vi "Drop Into MacroTree.vi"(0 "UI control refnums":T2, 1 "Index IN":i32, 5 "Source Tag":string, 7 "Source Text":string, 9 "Destination Tag":string, 11 "Error In":errorcluster, 12 "Drag Source":T1(ring)) -> (4 "Index OUT":i32, 14 "Any Error? OUT":bool, 15 "Error Out":errorcluster)   [LabVIEW 2012]
doc: "SciScan 1.2 160622"
uses:
  Custom Controls and Typedefs/Macro_MD_UI Control Refnums.ctl
  Custom Controls and Typedefs/Delete Button.ctl
  Custom Controls and Typedefs/Edit Button.ctl
  Custom Controls and Typedefs/Timing Estimate Cluster.ctl
  CommonResource VIs/Timing/Timing Indicator.ctl
  Custom Controls and Typedefs/Load from PSM Button.ctl
  CommonResource VIs/FormatTree&TableStyle_Commands.ctl
  Macro Loop Manager Module/SubVIs/Macro Execution and Timing_Commands.ctl
  SubVIs/FGV_MacroCore_Commands.ctl
panel:
  out "Specified tag is part of a Preset!":bool
  # "(hh:mm:ss)"
  # "(hh:mm:ss)"
  # "(hh:mm:ss)"
  # "(hh:mm:ss)"
  # "(hh:mm:ss)"
  # "(hh:mm:ss)"
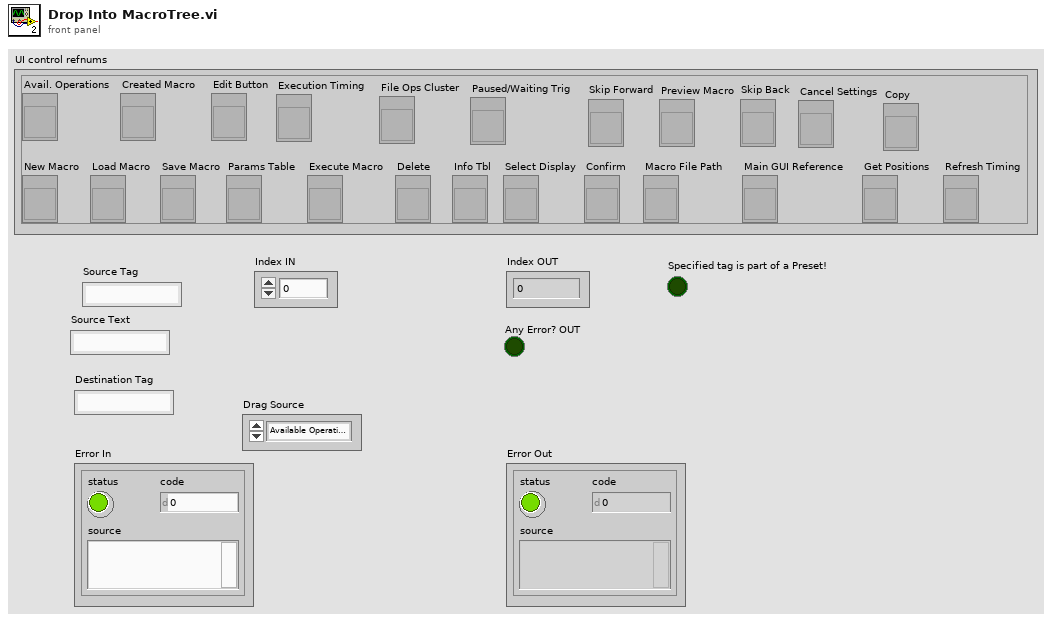
[diagram p1: front panel]
types:
  T1 = enum16{"Available Operations Tree", "Macro Tree"}
  T2 = typedef "Macro_MD_UI Control Refnums.ctl" = cluster{"Avail. Operations":refnum<vi>, "Created Macro":refnum<vi>, "Load Macro":refnum<vi>, "Save Macro":refnum<vi>, "Params Table":refnum<vi>, "Delete":refnum<vi>, "Edit Button":refnum<vi>, "Execute Macro":refnum<vi>, "Info Tbl":refnum<vi>, "Execution Timing":refnum<vi>, "Select Display":refnum<vi>, "File Ops Cluster":refnum<vi>, "Paused/Waiting Trig":refnum<vi>, "Confirm":refnum<vi>, "New Macro":refnum<vi>, "Preview Macro":refnum<vi>, "Skip Forward":refnum<vi>, "Skip Back":refnum<vi>, "Macro File Path":refnum<vi>, "Main GUI Reference":refnum<vi>, "Cancel Settings":refnum<vi>, "Get Positions":refnum<vi>, "Copy":refnum<vi>, "Refresh Timing":refnum<vi>}
  T3 = typedef "Macro Execution and Timing_Commands.ctl" = enum16{"Initialize (Update FGV & Rst Idx)", "Run", "EstimateTime", "Preview", "Update Macro array (Idx Unchanged)", "Update Index", "Clear Timing Info"}
  T4 = typedef "FormatTree&TableStyle_Commands.ctl" = enum16{"Colour Row", "Uncolour Row", "Bold Row", "Unbold Row", "Clear", "UpdateVisibleRows"}
  T5 = typedef "FGV_MacroCore_Commands.ctl" = enum16{"Initialize", "Get Array", "Load macro from file", "Insert Item", "Insert at End", "Edit Parameter String", "Delete instruction", "Move Items", "Save", "SaveAs", "UpdateInfoTable", "Edit Settings File", "New Macro", "Read Temp File", "Delete Multiple"}
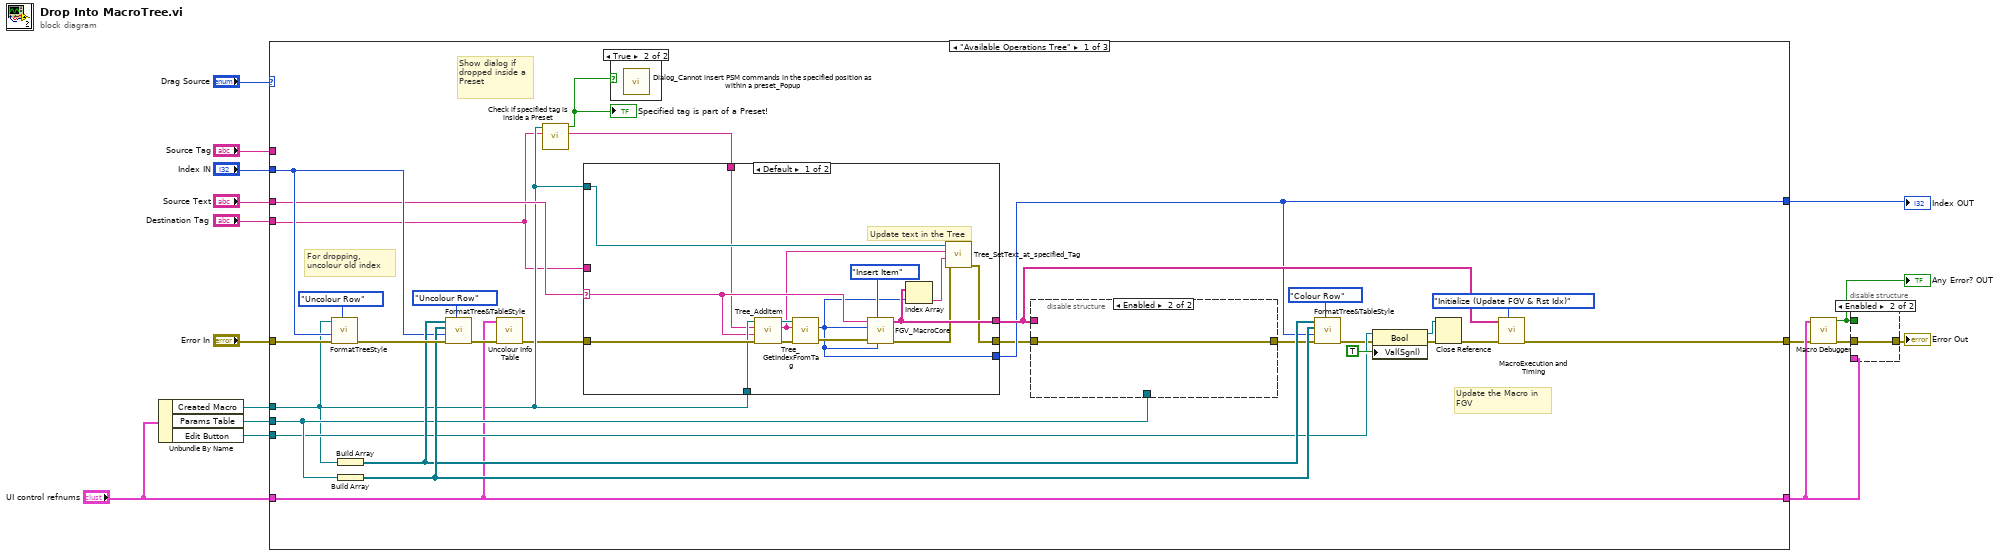
[diagram p0: block diagram]
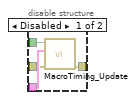
[diagram p2: hidden frame]
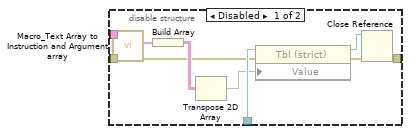
[diagram p4: hidden frame]
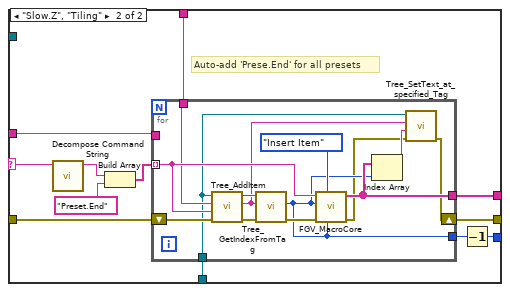
[diagram p5: hidden frame]
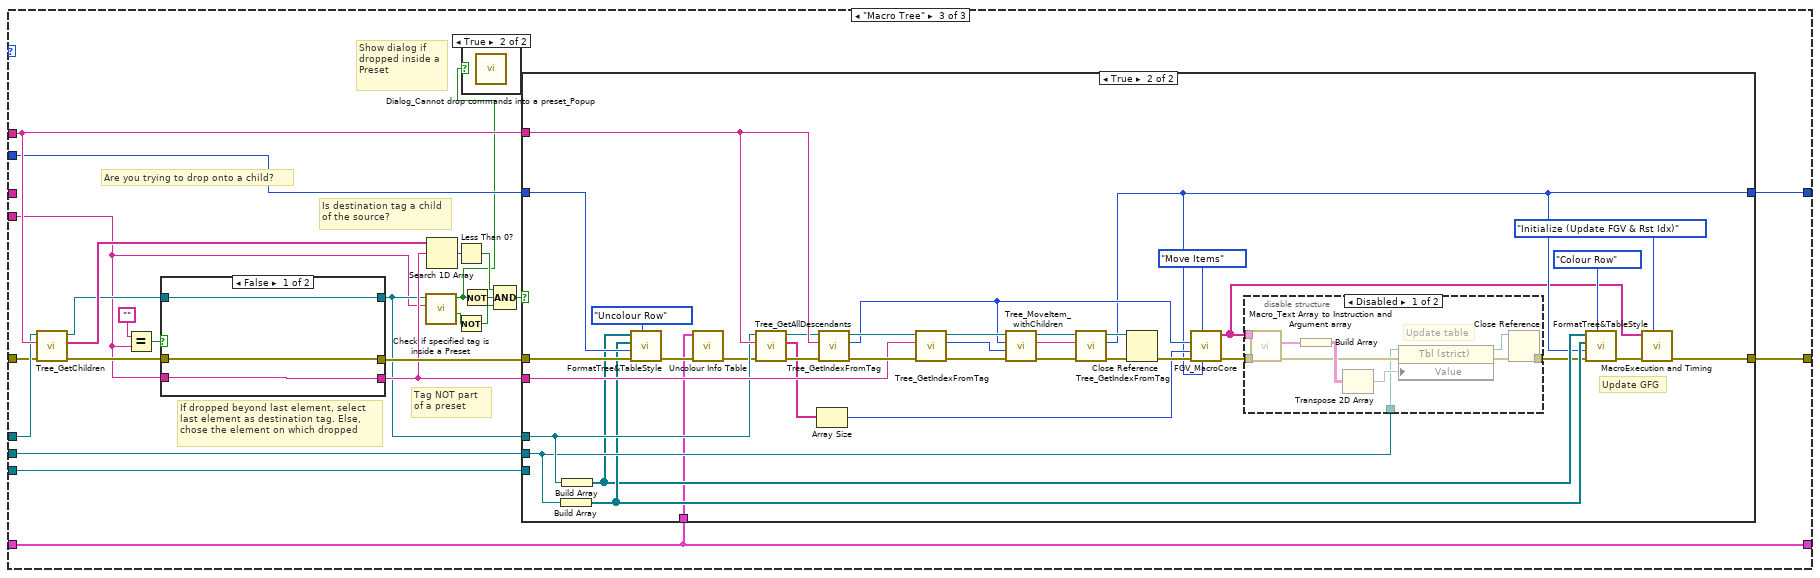
[diagram p7: hidden frame]
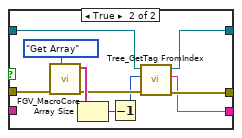
[diagram p9: hidden frame]
diagram:
  n1 = Unbundle By Name("UI control refnums") -> ("Created Macro"=w7:refnum<vi>, "Params Table"=w8:refnum<vi>, "Edit Button"=w9:refnum<vi>)
  n2 = case shown="\"Available Operations Tree\"" "Drag Source" {
    tunnel: "Source Tag" -> [_ _ w120]
    tunnel: "UI control refnums" -> [w26 w98 w109]
    tunnel: "Destination Tag" -> [w20 _ w107]
    tunnel: "Error In" -> [w32 w99 w113]
    tunnel: "Index IN" -> [w33 w100 w119]
    tunnel: [w24 w100 w118] -> w11
    tunnel: w9 -> [w34 _ w117]
    tunnel: w8 -> [w35 _ w116]
    tunnel: w7 -> [w22 _ w114]
    tunnel: "Source Text" -> [w23 _ _]
    tunnel: [w25 w99 w115] -> w3
    tunnel: [w26 w98 w109] -> w5
    frame "Available Operations Tree" {
      # "Show dialog if dropped inside a Preset"
      # "Update the Macro in \nFGV"
      # "For dropping, uncolour old index"
      n3 = call "FormatTreeStyle.vi"("Format Command"=FormatTree&TableStyle_Commands."Uncolour Row", "Error In"=w32, "Row Index"=w33, "Tree Refnum"=w22) -> ("Error Out"=w39:errorcluster)  [unwired: 7 in]
      n4 = Build Array(w22) -> (w37:refnum<vi>[])
      n5 = Build Array(w35) -> (w38:refnum<vi>[])
      n6 = call "FormatTree&TableStyle.vi"("Format Command"=FormatTree&TableStyle_Commands."Uncolour Row", "Error In"=w39, "Row Index"=w33, "Array of Table references"=w38, "Array of Tree references"=w37) -> ("Error Out"=w36:errorcluster)  [unwired: 6 in]
      n7 = call "Uncolour Info Table.vi"("Error In"=w36, "UI control refnums"=w26) -> ("Error Out"=w18:errorcluster)  [unwired: 9 in]
      n8 = call "Check if specified tag is inside a Preset.vi"("Tag to check"=w20, "Tree Refnum"=w22) -> ("Tag to add new item"=w19:string, "Specified tag is part of a Preset?"=w21:bool)  [unwired: 6 in, 2 out]
      "Specified tag is part of a Preset!" <- w21
      n9 = case shown="Default" w23 {
        selector: w23 -> [w65 w73]
        tunnel: [w58 w83] -> w17
        tunnel: w18 -> [w67 w82]
        tunnel: w20 -> [_ w75]
        tunnel: w22 -> [w66 w76]
        tunnel: [w64 w81] -> w27
        tunnel: [w63 w78] -> w24
        tunnel: w19 -> [w60 w74]
        tunnel: w22 -> [w61 _]
        frame Default {
          # "Update text in the Tree"
          n10 = call "Tree_AddItem.vi"("Error In"=w67, "NEW String"=w65, "Tag at add position"=w60, "Tree Refnum"=w66) -> ("Error Out"=w70:errorcluster, "Added Item Tag"=w57:string, "Tree Refnum OUT"=w68:refnum<vi>)  [unwired: 5 in]
          n11 = call "Tree_GetIndexFromTag.vi"("Error In"=w70, "Tag IN"=w57, "Tree Refnum IN"=w68) -> ("Error Out"=w69:errorcluster, "Index OUT"=w63:i32)  [unwired: 6 in, 1 out]
          n12 = call "FGV_MacroCore.vi"("Final Index"=w63, "MacroFGV_Commands"=FGV_MacroCore_Commands."Insert Item", "Error In"=w69, "Start Index"=w63, "Macro Command or Info (String)"=w65) -> ("Error Out"=w59:errorcluster, "Macro String Array"=w64:string[])  [unwired: 2 in, 3 out]
          n13 = Index Array(array=w64, index=w63) -> (element=w62:string)
          n14 = call "Tree_SetText_at_specified_Tag.vi"("Error In"=w59, "New String IN"=w62, "Tag (whose string to be edited)"=w57, "Tree Refnum IN"=w61) -> ("Error Out"=w58:errorcluster)  [unwired: 6 in, 1 out]
        }
        frame "Slow.Z", "Tiling" {
          # "Auto-add 'Prese.End' for all presets"
          n15 = call "Decompose Command String.vi"("Command IN"=w73) -> ("Action"=w72:string)  [unwired: 7 in, 3 out]
          n16 = Build Array(w72, "Preset.End" ("element")) -> (w77:string[])
          n17 = for {
            tunnel: w76 -> [w90]
            tunnel: [w88] -> w81
            tunnel: [w87] -> w79
            tunnel: w77 -> [w93] mode=indexing
            shift-right: [w84] -> w83
            shift-left: w82 -> [w94]
            tunnel: w75 -> [_]
            tunnel: w74 -> [w92]
            n18 = call "Tree_AddItem.vi"("Error In"=w94, "NEW String"=w93, "Tag at add position"=w92, "Tree Refnum"=w90) -> ("Error Out"=w96:errorcluster, "Added Item Tag"=w89:string, "Tree Refnum OUT"=w91:refnum<vi>)  [unwired: 5 in]
            n19 = call "Tree_GetIndexFromTag.vi"("Error In"=w96, "Tag IN"=w89, "Tree Refnum IN"=w91) -> ("Error Out"=w95:errorcluster, "Index OUT"=w87:i32)  [unwired: 6 in, 1 out]
            n20 = call "FGV_MacroCore.vi"("Final Index"=w87, "MacroFGV_Commands"=FGV_MacroCore_Commands."Insert Item", "Error In"=w95, "Start Index"=w87, "Macro Command or Info (String)"=w93) -> ("Error Out"=w85:errorcluster, "Macro String Array"=w88:string[])  [unwired: 2 in, 3 out]
            n21 = Index Array(array=w88, index=w87) -> (element=w86:string)
            n22 = call "Tree_SetText_at_specified_Tag.vi"("Error In"=w85, "New String IN"=w86, "Tag (whose string to be edited)"=w89, "Tree Refnum IN"=w90) -> ("Error Out"=w84:errorcluster)  [unwired: 6 in, 1 out]
          }
          n23 = Decrement(x=w79) -> (x-1=w78:i32)
        }
      }
      n24 = case shown="True" w21 {
        frame False {
        }
        frame True {
          n25 = call "Dialog_Cannot insert PSM commands in the specified position as within a preset_Popup.vi"() -> ()  [unwired: 11 in, 1 out]
        }
      }
      n26 = disable-structure shown="Enabled" {
        disable-tunnel: w17 -> [w55 w56]
        disable-tunnel: w35 -> [w54 _]
        disable-tunnel: [w53 w56] -> w30
        disable-tunnel: w27 -> [w52 _]
        frame Disabled {
          n27 = call "Macro_Text Array to Instruction and Argument array.vi"("Error In"=w55, "Macro Array IN"=w52) -> ("Error Out"=w49:errorcluster, "Argument List (Txt)"=w48:string[])  [unwired: 7 in, 1 out]
          n28 = Build Array(w48) -> (w51:string[][])
          n29 = Transpose 2D Array(2D array=w51) -> (transposed array=w50:string[][])
          n30 = property class="Tbl (strict)"(reference=w54, error in=w49, "Value"=w50) -> (reference out=w46:refnum<vi>, error out=w47:errorcluster)
          n31 = Close Reference(reference=w46, error in (no error)=w47) -> (error out=w53:errorcluster)
        }
        frame Enabled {
        }
      }
      n32 = call "FormatTree&TableStyle.vi"("Format Command"=FormatTree&TableStyle_Commands."Colour Row", "Error In"=w30, "Row Index"=w24, "Array of Table references"=w38, "Array of Tree references"=w37) -> ("Error Out"=w31:errorcluster)  [unwired: 6 in]
      n33 = property class="Bool"(reference=w34, error in=w31, "Val(Sgnl)"=TRUE) -> (reference out=w43:refnum<vi>, error out=w44:errorcluster)
      n34 = Close Reference(reference=w43, error in (no error)=w44) -> (error out=w28:errorcluster)
      n35 = call "MacroExecution and Timing.vi"("MacroExecution and Timing Command"=Macro_Execution_and_Timing_Commands."Initialize (Update FGV & Rst Idx)" ("MacroExecution Command"), "Error In"=w28, "Macro IN"=w27) -> ("Error Out"=w25:errorcluster)  [unwired: 3 in, 5 out]
    }
    frame Default {
    }
    frame "Macro Tree" {
      # "Show dialog if dropped inside a Preset"
      # "Tag NOT part of a preset"
      # "Is destination tag a child\nof the source?"
      # "Are you trying to drop onto a child?"
      # "If dropped beyond last element, select\nlast element as destination tag. Else,\nchose the element on which dropped"
      n36 = call "Tree_GetChildren.vi"("Error In"=w113, "Parent Tag"=w120, "Tree Refnum IN"=w114) -> ("Error Out"=w112:errorcluster, "Children Tags"=w125:string[], "Tree Refnum OUT"=w111:refnum<vi>)  [unwired: 6 in]
      n37 = Equal?(x="", y=w107) -> (x = y?=w122:bool)
      n38 = case shown="False" w122 {
        tunnel: w112 -> [w128 w136]
        tunnel: w111 -> [w126 w134]
        tunnel: [w128 w131] -> w121
        tunnel: [w127 w130] -> w110
        tunnel: w107 -> [w127 _]
        tunnel: [w126 w129] -> w108
        frame False {
        }
        frame True {
          n39 = call "FGV_MacroCore.vi"("MacroFGV_Commands"=FGV_MacroCore_Commands."Get Array", "Error In"=w136) -> ("Error Out"=w135:errorcluster, "Macro String Array"=w137:string[])  [unwired: 5 in, 3 out]
          n40 = Array Size(array=w137) -> (size(s)=w133:i32)
          n41 = Decrement(x=w133) -> (x-1=w132:i32)
          n42 = call "Tree_GetTag FromIndex.vi"("Error In"=w135, "Index IN"=w132, "Tree Refnum IN"=w134) -> ("Error Out"=w131:errorcluster, "Tag OUT"=w130:string, "Tree Refnum OUT"=w129:refnum<vi>)  [unwired: 6 in]
        }
      }
      n43 = call "Check if specified tag is inside a Preset.vi"("Tag to check"=w107, "Tree Refnum"=w108) -> ("Specified Tag is a Preset command?"=w102:bool, "Specified tag is part of a Preset?"=w101:bool)  [unwired: 6 in, 2 out]
      n44 = Search 1D Array(1D array=w125, element=w110) -> (index of element=w123:i32)  [unwired: 1 in]
      n45 = Less Than 0?(x=w123) -> (x < 0?=w106:bool)
      n46 = Not(x=w102) -> (.not. x?=w103:bool)
      n47 = case shown="True" w101 {
        frame False {
        }
        frame True {
          n48 = call "Dialog_Cannot drop commands into a preset_Popup.vi"() -> ()  [unwired: 11 in, 1 out]
        }
      }
      n49 = Not(x=w101) -> (.not. x?=w104:bool)
      n50 = Compound Arithmetic op=AND(w106, w104, w103) -> (w105:bool)
      n51 = case shown="True" w105 {
        tunnel: w121 -> [w139 w153]
        tunnel: w110 -> [_ w173]
        tunnel: w120 -> [_ w166]
        tunnel: w119 -> [w140 w154]
        tunnel: [w140 w149] -> w118
        tunnel: w116 -> [_ w155]
        tunnel: [w139 w141] -> w115
        tunnel: w108 -> [_ w156]
        tunnel: w109 -> [_ w146]
        tunnel: w117 -> [_ _]
        frame False {
        }
        frame True {
          # "Update GFG"
          n52 = Build Array(w155) -> (w151:refnum<vi>[])
          n53 = Build Array(w156) -> (w150:refnum<vi>[])
          n54 = call "FormatTree&TableStyle.vi"("Format Command"=FormatTree&TableStyle_Commands."Uncolour Row", "Error In"=w153, "Row Index"=w154, "Array of Table references"=w151, "Array of Tree references"=w150) -> ("Error Out"=w148:errorcluster)  [unwired: 6 in]
          n55 = call "Uncolour Info Table.vi"("Error In"=w148, "UI control refnums"=w146) -> ("Error Out"=w147:errorcluster)  [unwired: 9 in]
          n56 = call "Tree_GetAllDescendants.vi"("Error In"=w147, "Tag"=w166, "Tree Refnum IN"=w156) -> ("Error Out"=w165:errorcluster, "All Descendants"=w163:string[], "Tree Refnum OUT"=w164:refnum<vi>)  [unwired: 6 in]
          n57 = Array Size(array=w163) -> (size(s)=w159:i32)
          n58 = call "Tree_GetIndexFromTag.vi"("Error In"=w165, "Tag IN"=w166, "Tree Refnum IN"=w164) -> ("Error Out"=w176:errorcluster, "Index OUT"=w160:i32, "Tree Refnum OUT"=w177:refnum<vi>)  [unwired: 6 in]
          n59 = call "Tree_GetIndexFromTag.vi"("Error In"=w176, "Tag IN"=w173, "Tree Refnum IN"=w177) -> ("Error Out"=w175:errorcluster, "Index OUT"=w172:i32, "Tree Refnum OUT"=w174:refnum<vi>)  [unwired: 6 in]
          n60 = call "Tree_MoveItem_withChildren.vi"("Error In"=w175, "End Index"=w172, "Start Index"=w160, "Tree Refnum IN"=w174) -> ("Error Out"=w170:errorcluster, "Moved Tag"=w168:string, "Tree Refnum OUT"=w169:refnum<vi>)  [unwired: 5 in]
          n61 = call "Tree_GetIndexFromTag.vi"("Error In"=w170, "Tag IN"=w168, "Tree Refnum IN"=w169) -> ("Error Out"=w171:errorcluster, "Index OUT"=w149:i32, "Tree Refnum OUT"=w167:refnum<vi>)  [unwired: 6 in]
          n62 = Close Reference(reference=w167, error in (no error)=w171) -> (error out=w161:errorcluster)
          n63 = call "FGV_MacroCore.vi"("Final Index"=w149, "MacroFGV_Commands"=FGV_MacroCore_Commands."Move Items", "Error In"=w161, "Length"=w159, "Start Index"=w160) -> ("Error Out"=w158:errorcluster, "Macro String Array"=w143:string[])  [unwired: 2 in, 3 out]
          n64 = disable-structure shown="Disabled" {
            disable-tunnel: w158 -> [w183 _]
            disable-tunnel: w155 -> [w180 _]
            disable-tunnel: [w179 _] -> w145
            disable-tunnel: w143 -> [w178 _]
            frame Disabled {
              # "Update table"
              n65 = call "Macro_Text Array to Instruction and Argument array.vi"("Error In"=w183, "Macro Array IN"=w178) -> ("Error Out"=w182:errorcluster, "Argument List (Txt)"=w181:string[])  [unwired: 7 in, 1 out]
              n66 = Build Array(w181) -> (w186:string[][])
              n67 = Transpose 2D Array(2D array=w186) -> (transposed array=w185:string[][])
              n68 = property class="Tbl (strict)"(reference=w180, error in=w182, "Value"=w185) -> (reference out=w184:refnum<vi>, error out=w187:errorcluster)
              n69 = Close Reference(reference=w184, error in (no error)=w187) -> (error out=w179:errorcluster)
            }
            frame Enabled {
            }
          }
          n70 = call "FormatTree&TableStyle.vi"("Format Command"=FormatTree&TableStyle_Commands."Colour Row", "Error In"=w145, "Row Index"=w149, "Array of Table references"=w151, "Array of Tree references"=w150) -> ("Error Out"=w142:errorcluster)  [unwired: 6 in]
          n71 = call "MacroExecution and Timing.vi"("MacroExecution and Timing Command"=Macro_Execution_and_Timing_Commands."Initialize (Update FGV & Rst Idx)" ("MacroExecution Command"), "Error In"=w142, "Macro IN"=w143) -> ("Error Out"=w141:errorcluster)  [unwired: 3 in, 5 out]
        }
      }
    }
  }
  "Index OUT" <- w11
  n72 = call "Macro Debugger.vi"("Error In"=w3, "UI control refnums"=w5) -> ("Error Out"=w2:errorcluster, "Any Error?"=w4:bool)  [unwired: 8 in]
  "Any Error? OUT" <- w4
  n73 = disable-structure shown="Enabled" {
    disable-tunnel: w5 -> [w191 _]
    disable-tunnel: w4 -> [w190 _]
    disable-tunnel: w2 -> [w189 w192]
    disable-tunnel: [w188 w192] -> w1
    frame Disabled {
      n74 = call "MacroTiming_Update.vi"("error in (no error)"=w189, "UI control refnums"=w191, "Macro Error IN?"=w190) -> ("error out"=w188:errorcluster)  [unwired: 8 in]
    }
    frame Enabled {
    }
  }
  "Error Out" <- w1
